vi "DisableOutput.vi"(8 "error in (no error)":errorcluster, 11 "Pod Drive in":refnum<class "Pod Drive.lvclass">) -> (0 "error out":errorcluster, 3 "Pod Drive out":refnum<class "Pod Drive.lvclass">)   [LabVIEW 2019, in "DriveOld.lvlib" / "Pod Drive.lvclass"]
doc: "The Talons store setpoints even after disabling the robot so this VI goes into disabled.VI and sets the talons output to zero"
uses:
  Pod Drive.lvclass
  <vilib>/Rock Robotics/WPI/ThirdParty/Phoenix-LabVIEW/Motor Controller/Controls/CTRE_Phoenix_MotorControl_ControlMode.ctl
  Pod Drive.lvclass/Pod Drive.ctl
  Drive.lvclass
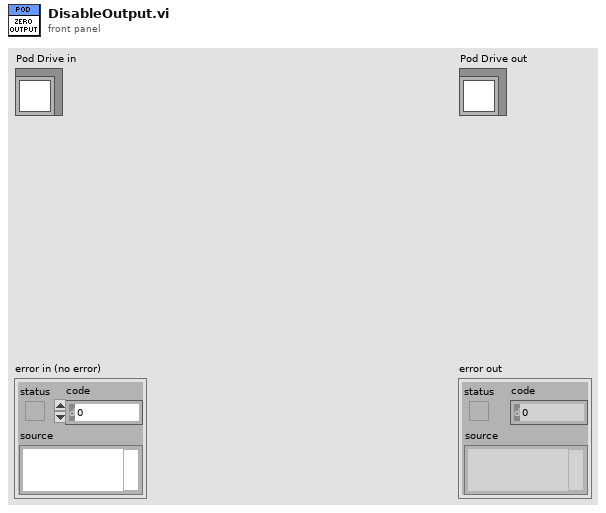
[diagram p1: front panel]
types:
  T1 = typedef "CTRE_Phoenix_MotorControl_ControlMode.ctl" = u16
  T2 = typedef "WPI_MotorControlDeviceRef.ctl" = cluster{"DeviceStatus":errorcluster, "Type":T3, "PWM":cluster{"PWM Channel":T4, "DeadBand":T5}, "CAN":cluster{"Device Number":u8, "SetOutput VI Ref":variant, "GetOutput VI Ref":variant, "Enable VI Ref":variant, "Disable VI Ref":variant, "Data":variant}, "Invert":bool, "DIO PWM":cluster{"PWM \"Enable\" Channel":T4, "DIOChannel":T6, "PWM Rate":dbl}}
  T3 = typedef "WPI_MotorControlType.ctl" = enum16{"PWM", "CAN", "DIO PWM"}
  T4 = typedef "FPGA_DIOPWMChannel.ctl" = enum8{"PWM 0", "PWM 1", "PWM 2", "PWM 3", "PWM 4", "PWM 5", "PWM 6", "PWM 7", "PWM 8", "PWM 9", "PWM MXP 0", "PWM MXP 1", "PWM MXP 2", "PWM MXP 3", "PWM MXP 4", "PWM MXP 5", "PWM MXP 6", "PWM MXP 7", "PWM MXP 8", "PWM MXP 9", "Invalid"}
  T5 = typedef "WPI_PWMDeadband.ctl" = cluster{"Name":string, "maxPositivePwm":i32, "minPositivePwm":i32, "centerPwm":i32, "maxNegativePwm":i32, "minNegativePwm":i32, "angularRange":u16}
  T6 = typedef "FPGA_DIOChannel.ctl" = enum8{"DIO 0", "DIO 1", "DIO 2", "DIO 3", "DIO 4", "DIO 5", "DIO 6", "DIO 7", "DIO 8", "DIO 9", "DIO MXP 0", "DIO MXP 1", "DIO MXP 2", "DIO MXP 3", "DIO MXP 4", "DIO MXP 5", "DIO MXP 6", "DIO MXP 7", "DIO MXP 8", "DIO MXP 9", "DIO MXP 10", "DIO MXP 11", "DIO MXP 12", "DIO MXP 13", "DIO MXP 14", "DIO MXP 15", "SPI Port CS1", "SPI Port CS2", "SPI Port CS3", "SPI Port MISO", "SPI Port MOSI", "Invalid"}
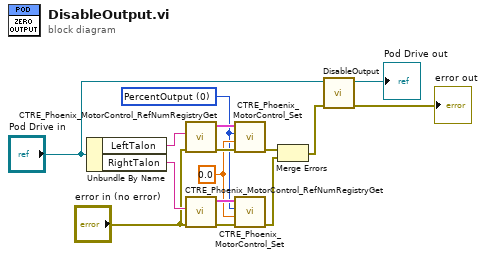
[diagram p0: block diagram]
diagram:
  w6 = 0.0 ("Output")
  w5 = T1 0 items=["PercentOutput"=0, "Position"=1, "Velocity"=2, "Current"=3, "Follower"=5, "MotionProfile"=6, "MotionMagic"=7, "MotionProfileArc"=10, "Disabled"=15] ("Control Mode")
  n1 = Unbundle By Name("Pod Drive in") -> ("LeftTalon"=w7:string, "RightTalon"=w8:string)
  n2 = call <vilib>:"CTRE_Phoenix_MotorControl_RefNumRegistryGet.vi"("error in (no error)"="error in (no error)", "refnum name"=w7) -> ("error out"=w12:errorcluster, "PhoenixMotorControlDevRef"=w11:T2)  [unwired: 8 in]
  n3 = call <vilib>:"CTRE_Phoenix_MotorControl_RefNumRegistryGet.vi"("error in (no error)"="error in (no error)", "refnum name"=w8) -> ("error out"=w10:errorcluster, "PhoenixMotorControlDevRef"=w9:T2)  [unwired: 8 in]
  n4 = call <vilib>:"CTRE_Phoenix_MotorControl_Set.vi"("error in (no error)"=w12, "Output"=w6, "Control Mode"=w5, "PhoenixMotorControlDevRef"=w11) -> ("error out"=w3:errorcluster)  [unwired: 6 in, 1 out]
  n5 = call <vilib>:"CTRE_Phoenix_MotorControl_Set.vi"("error in (no error)"=w10, "Output"=w6, "Control Mode"=w5, "PhoenixMotorControlDevRef"=w9) -> ("error out"=w2:errorcluster)  [unwired: 6 in, 1 out]
  n6 = Merge Errors(w3, w2) -> (w1:errorcluster)
  n7 = call-parent "DisableOutput.vi"("error in (no error)"=w1, "Drive in"="Pod Drive in") -> ("error out"=→"error out":errorcluster, "Drive out"=→"Pod Drive out":refnum<class "Pod Drive.lvclass">)  [unwired: 8 in]
